vi "Read Buffer Statistics.vi"(0 "VISA resource name":refnum<visa-resource-name>, 11 "error in (no error)":errorcluster) -> (3 "Mean":dbl, 4 "VISA resource name out":refnum<visa-resource-name>, 6 "Maximum":dbl, 8 "Minimum":dbl, 10 "Standard Deviation":dbl, 14 "Reading Count":i32, 15 "error out":errorcluster)   [LabVIEW 2021, in "Keithley 648X Series.lvlib"]
doc: "Reads the statistical properties of the data buffer."
uses:
  <instrlib>/Keithley 648X Series/Keithley 648X Series.lvlib
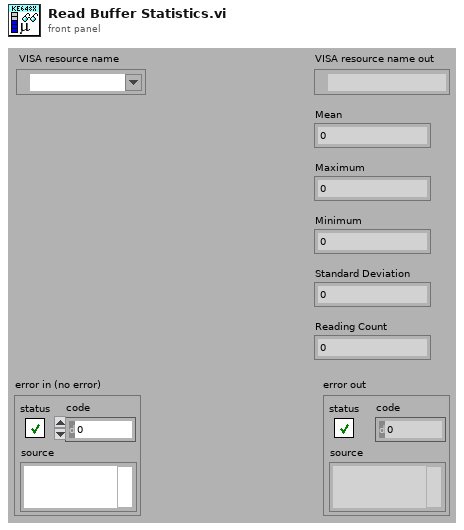
[diagram p1: front panel]
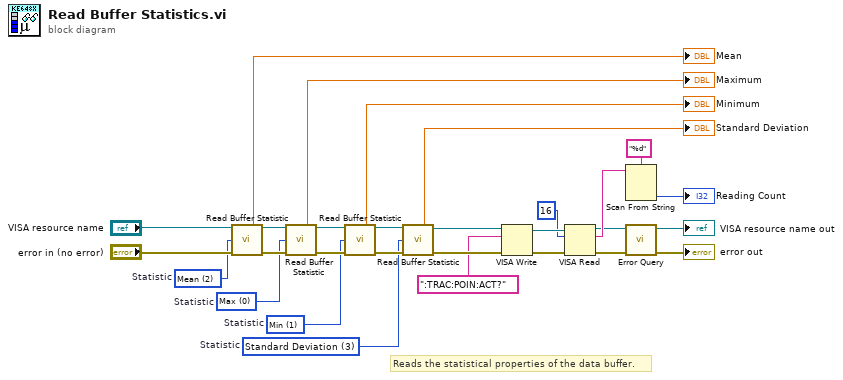
[diagram p0: block diagram]
diagram:
  w18 = u16 3 items=["Max", "Min", "Mean", "Standard Deviation", "Peak to Peak"]  # Statistic
  w19 = u16 1 items=["Max", "Min", "Mean", "Standard Deviation", "Peak to Peak"]  # Statistic
  w20 = u16 0 items=["Max", "Min", "Mean", "Standard Deviation", "Peak to Peak"]  # Statistic
  w21 = u16 2 items=["Max", "Min", "Mean", "Standard Deviation", "Peak to Peak"]  # Statistic
  # "Reads the statistical properties of the data buffer."
  n1 = call <instrlib>:"Read Buffer Statistic.vi"("VISA resource name"="VISA resource name", "Statistic (0: Max)"=w21, "error in (no error)"="error in (no error)") -> ("Buffer Statistic"=→"Mean":dbl, "VISA resource name out"=w25:refnum<visa-resource-name>, "error out"=w24:errorcluster)  [unwired: 10 in]
  n2 = call <instrlib>:"Read Buffer Statistic.vi"("VISA resource name"=w25, "Statistic (0: Max)"=w20, "error in (no error)"=w24) -> ("Buffer Statistic"=→"Maximum":dbl, "VISA resource name out"=w22:refnum<visa-resource-name>, "error out"=w23:errorcluster)  [unwired: 10 in]
  n3 = call <instrlib>:"Read Buffer Statistic.vi"("VISA resource name"=w22, "Statistic (0: Max)"=w19, "error in (no error)"=w23) -> ("Buffer Statistic"=→"Minimum":dbl, "VISA resource name out"=w29:refnum<visa-resource-name>, "error out"=w28:errorcluster)  [unwired: 10 in]
  n4 = call <instrlib>:"Read Buffer Statistic.vi"("VISA resource name"=w29, "Statistic (0: Max)"=w18, "error in (no error)"=w28) -> ("Buffer Statistic"=→"Standard Deviation":dbl, "VISA resource name out"=w12:refnum<visa-resource-name>, "error out"=w13:errorcluster)  [unwired: 10 in]
  n5 = VISA Write(VISA resource name=w12, write buffer=":TRAC:POIN:ACT?", error in (no error)=w13) -> (VISA resource name out=w10:refnum<visa-resource-name>, error out=w11:errorcluster)  [unwired: 1 out]
  n6 = VISA Read(VISA resource name=w10, byte count=u32 16, error in (no error)=w11) -> (VISA resource name out=w2:refnum<visa-resource-name>, read buffer=w6:string, error out=w5:errorcluster)  [unwired: 1 out]
  n7 = Scan From String(format string="%d", input string=w6) -> (output 1=→"Reading Count":i32)  [unwired: 3 in, 3 out]
  n8 = call <instrlib>:"Error Query.vi"("error in (no error)"=w5, "VISA resource name"=w2) -> ("error out"=→"error out":errorcluster, "VISA resource name out"=→"VISA resource name out":refnum<visa-resource-name>)  [unwired: 6 in, 2 out]
